vi "Get Section.vi"(11 "Optional Objects in":refnum<class "Optional Objects.lvclass">) -> (2 "Section":string, 3 "Optional Objects out":refnum<class "Optional Objects.lvclass">)   [LabVIEW 2024, in "Optional Objects.lvclass"]
uses:
  Optional Objects.lvclass
  Optional Objects.lvclass/Optional Objects.ctl
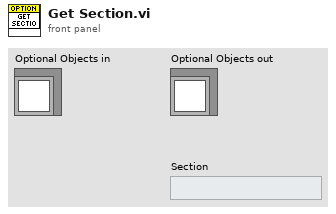
[diagram p1: front panel]
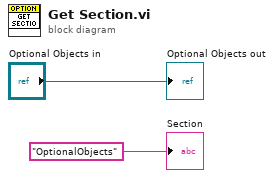
[diagram p0: block diagram]
diagram:
  "Optional Objects out" <- "Optional Objects in"
  "Section" <- "OptionalObjects" ("Section")
